vi "Servo.vi"() -> ()   [LabVIEW 2025]
doc: "This example shows how to set and read the angle of a servo.\n\nThis example expects a USB cable connected from your development PC to the Type B USB Jack (next to the power input) on the roboRIO.\n\nThis example requires the Driver Station to be running with Teleoperated Enabled."
uses:
  <vilib>/Rock Robotics/SystemInterfaces/DIO/FPGA_DIOPWMChannel.ctl
panel:
  in  "PWM Channel":T1=enum."PWM 7"
  in  "Desired Angle":i32(knob) scale=0.0..170.0
  out "Current Angle":u16(knob) scale=0.0..170.0
  in  "stop":bool
  # "Set this input before running."
  # "This can be set while running."
  # "This example requires the Driver Station to be running with Teleoperated Enabled."
  # "PWM cable"
  # "This shows wiring for a HiTEC servo.  The black wire connects to ground (-). The red wire connects to power (V). The white or yellow wire connects to signal (S)."
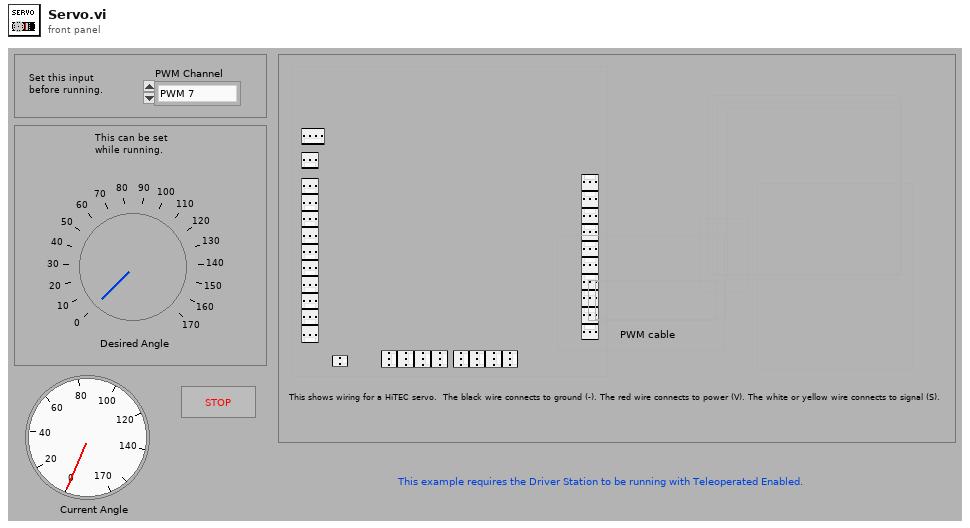
[diagram p1: front panel]
types:
  T1 = typedef "FPGA_DIOPWMChannel.ctl" = enum8{"PWM 0", "PWM 1", "PWM 2", "PWM 3", "PWM 4", "PWM 5", "PWM 6", "PWM 7", "PWM 8", "PWM 9", "PWM MXP 0", "PWM MXP 1", "PWM MXP 2", "PWM MXP 3", "PWM MXP 4", "PWM MXP 5", "PWM MXP 6", "PWM MXP 7", "PWM MXP 8", "PWM MXP 9", "Invalid"}
  T2 = typedef "WPI_ServoDeviceRef.ctl" = cluster{"DeviceStatus":errorcluster, "PWM Channel":T1, "DeadBand":T3}
  T3 = typedef "WPI_PWMDeadband.ctl" = cluster{"Name":string, "maxPositivePwm":i32, "minPositivePwm":i32, "centerPwm":i32, "maxNegativePwm":i32, "minNegativePwm":i32, "angularRange":u16}
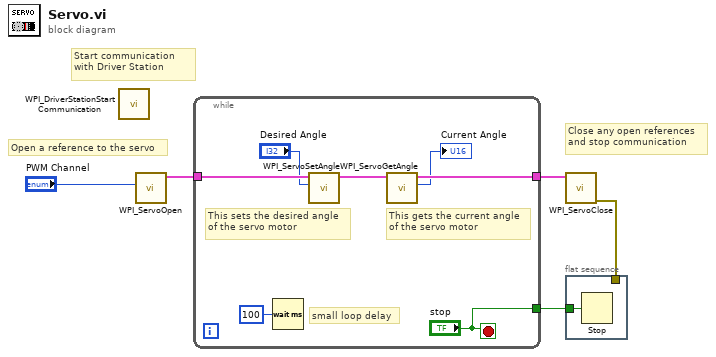
[diagram p0: block diagram]
diagram:
  # "Close any open references\nand stop communication"
  # "Start communication with Driver Station"
  # "Open a reference to the servo"
  n1 = call <vilib>:"WPI_DriverStationStart Communication.vi"() -> ()  [unwired: 3 in, 9 out]
  n2 = call <vilib>:"WPI_ServoOpen.vi"("PWM Channel"="PWM Channel") -> ("ServoDeviceRef"=w5:T2)  [unwired: 3 in, 7 out]
  n3 = while {
    tunnel: w5 -> [w12]
    tunnel: [w10] -> w4
    tunnel: ["stop"] -> w2
    stop <- "stop" stop-if-true
    # "small loop delay"
    # "This gets the current angle\nof the servo motor"
    # "This sets the desired angle \nof the servo motor"
    n4 = Wait (ms)(milliseconds to wait=u32 100) -> ()  [unwired: 1 out]
    n5 = call <vilib>:"WPI_ServoSetAngle.vi"("Angle"="Desired Angle", "ServoDeviceRef"=w12) -> ("ServoDeviceRef"=w11:T2)  [unwired: 1 in, 8 out]
    n6 = call <vilib>:"WPI_ServoGetAngle.vi"("ServoDeviceRef"=w11) -> ("ServoDeviceRef"=w10:T2, "Angle"=→"Current Angle":u16)  [unwired: 1 in, 7 out]
  }
  n7 = call <vilib>:"WPI_ServoClose.vi"("ServoDeviceRef"=w4) -> ("error out"=w1:errorcluster)  [unwired: 1 in, 9 out]
  n8 = flat-sequence {
    tunnel: w2 -> [w13]
    tunnel: w1 -> [_]
    frame #0 {
      n9 = Stop(stop? (T)=w13) -> ()
    }
  }
